vi "CRYFlatten Multimeter.vi"(11 "Voltmeter Settings":T1={"Ave/Max/Min"=0, "Level"=0, "Channel"=0, "Signal Type"="None", "Weighting"="None", "Applay Correction"=FALSE, "lin/exp avg"=0, "rec time (sec)"=0.0009999999999998899, "Average Time (Sec)"=0.0009999999999998899, "Lin Display Prefs"="%#_6p", "dB Display Prefs"="%.1f", "Time Weighting"=0, "Display"=0}) -> (3 "Flat Voltmeter setup":string)   [LabVIEW 2013]
uses:
  Typedef Control/CRYMultimeter.ctl
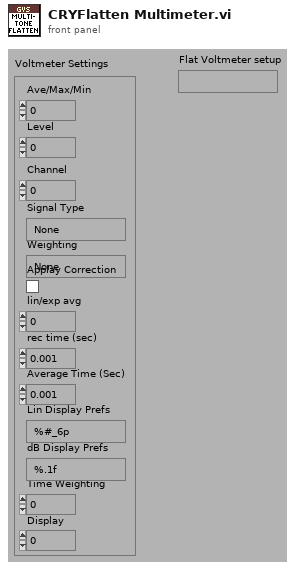
[diagram p1: front panel]
types:
  T1 = typedef "CRYMultimeter.ctl" = cluster{"Ave/Max/Min":i32, "Level":i32, "Channel":i32, "Signal Type":string, "Weighting":string, "Applay Correction":bool, "lin/exp avg":u16, "rec time (sec)":dbl, "Average Time (Sec)":dbl, "Lin Display Prefs":string, "dB Display Prefs":string, "Time Weighting":u16, "Display":u16}
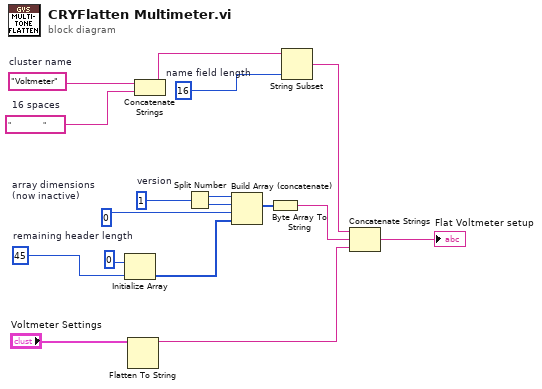
[diagram p0: block diagram]
diagram:
  w4 = u8 0  # array dimensions (now inactive)
  w7 = 16  # name field length
  w8 = "                "  # 16 spaces
  w9 = "Voltmeter"  # cluster name
  w13 = 45  # remaining header length
  w17 = u16 1  # version
  n1 = Initialize Array(u8 0, w13) -> (w10:u8[])
  n2 = Flatten To String(anything="Voltmeter Settings") -> (data string=w3:string)  [unwired: 1 in, 4 out]
  n3 = Concatenate Strings(w9, w8) -> (w6:string)
  n4 = Split Number(x=w17) -> (hi(x)=w16:u8, lo(x)=w15:u8)
  n5 = Build Array (concatenate)(w16, w15, w4, w10) -> (w12:u8[])
  n6 = Byte Array To String(unsigned byte array=w12) -> (string=w11:string)
  n7 = String Subset(string=w6, length (rest)=w7) -> (substring=w5:string)  [unwired: 1 out]
  n8 = Concatenate Strings(w5, w11, w3) -> (→"Flat Voltmeter setup":string)
